vi "PrgFGV.vi"(9 "Index":i8, 10 "Action":T1(ring), 11 "CYL in":refnum<class "Cycle.lvclass">) -> (1 "PRG out":refnum<class "Cycle.lvclass">[](array[class]), 2 "Size":i8, 3 "CYL out":refnum<class "Cycle.lvclass">)   [LabVIEW 2012, in "StimulCtrls.lvlib"]
uses:
  StimulCtrls.lvlib
  CYL/Cycle.lvclass
panel:
  # "Functional global variable to save PRG"
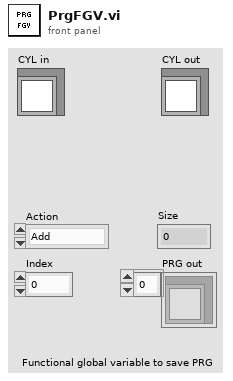
[diagram p1: front panel]
types:
  T1 = enum16{"Add", "New", "Del", "Update", "Get", "Initial", "GetSize"}
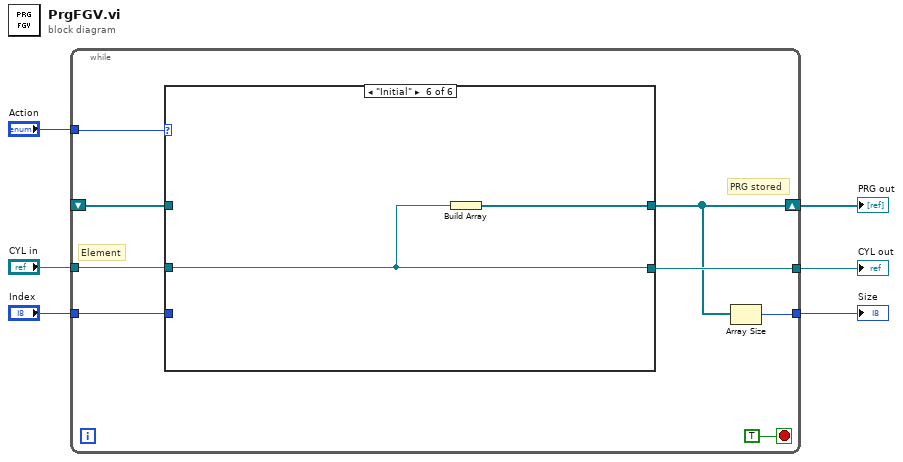
[diagram p0: block diagram]
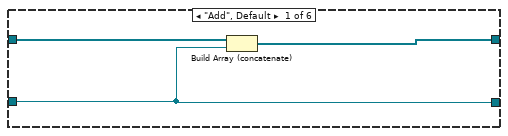
[diagram p2: hidden frame]
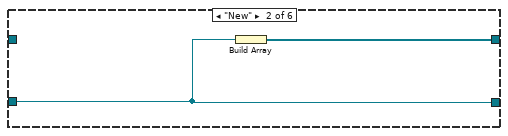
[diagram p3: hidden frame]
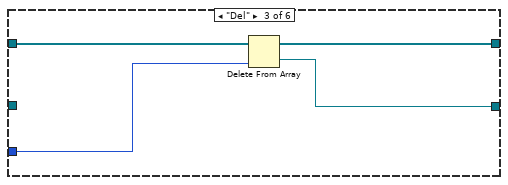
[diagram p4: hidden frame]
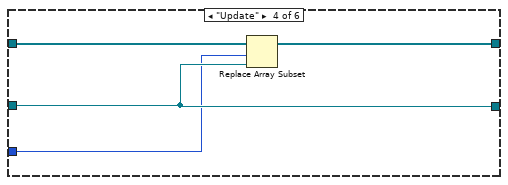
[diagram p5: hidden frame]
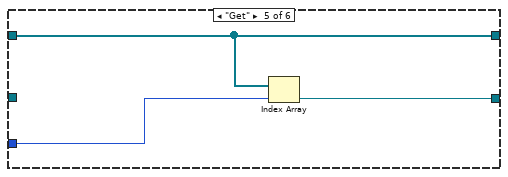
[diagram p6: hidden frame]
diagram:
  n1 = while {
    tunnel: "CYL in" -> [w13]
    shift-right: [w9] -> w2
    shift-left: _ -> [w12]
    tunnel: [w11] -> w1
    tunnel: [w10] -> w6
    tunnel: "Index" -> [w8]
    tunnel: "Action" -> [w7]
    stop <- TRUE stop-if-true
    # "PRG stored"
    # "Element"
    n2 = case shown="\"Initial\"" w7 {
      tunnel: w13 -> [w15 w18 _ w25 _ w31]
      tunnel: w12 -> [w17 _ w23 w27 w30 _]
      tunnel: [w16 w19 w21 w26 w30 w32] -> w9
      tunnel: w8 -> [_ _ w22 w24 w29 _]
      tunnel: [w15 w18 w20 w25 w28 w31] -> w11
      frame "Add", Default {
        n3 = Build Array (concatenate)(w17, w15) -> (w16:refnum<class "Cycle.lvclass">[])
      }
      frame "New" {
        n4 = Build Array(w18) -> (w19:refnum<class "Cycle.lvclass">[])
      }
      frame "Del" {
        n5 = Delete From Array(array=w23, index=w22) -> (deleted portion=w20:refnum<class "Cycle.lvclass">, array with subset deleted=w21:refnum<class "Cycle.lvclass">[])  [unwired: 1 in]
      }
      frame "Update" {
        n6 = Replace Array Subset(array=w27, new element=w25, index=w24) -> (w26:refnum<class "Cycle.lvclass">[])
      }
      frame "Get" {
        n7 = Index Array(array=w30, index=w29) -> (element=w28:refnum<class "Cycle.lvclass">)
      }
      frame "Initial" {
        n8 = Build Array(w31) -> (w32:refnum<class "Cycle.lvclass">[])
      }
    }
    n9 = Array Size(array=w9) -> (size(s)=w10:i32)
  }
  "Size" <- w6
  "PRG out" <- w2
  "CYL out" <- w1
